vi "Acquire Image.vi"(8 "error in (no error)":errorcluster, 11 "Simulated Camera in":refnum<class "Simulated Camera.lvclass">) -> (0 "error out":errorcluster, 3 "Simulated Camera out":refnum<class "Simulated Camera.lvclass">)   [LabVIEW 2019, in "Simulated Camera.lvclass"]
uses:
  Simulated Camera.lvclass
  Simulated Camera.lvclass/Simulated Camera.ctl
  <vilib>/numeric/Random Number (Range) U64.vi
  <vilib>/numeric/sub_Random U32.vi
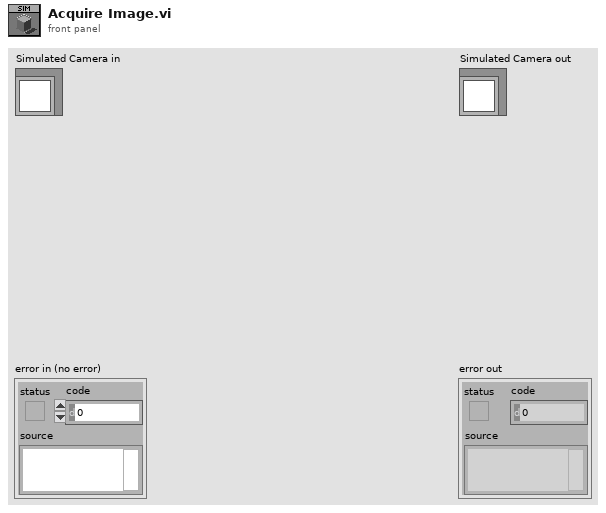
[diagram p1: front panel]
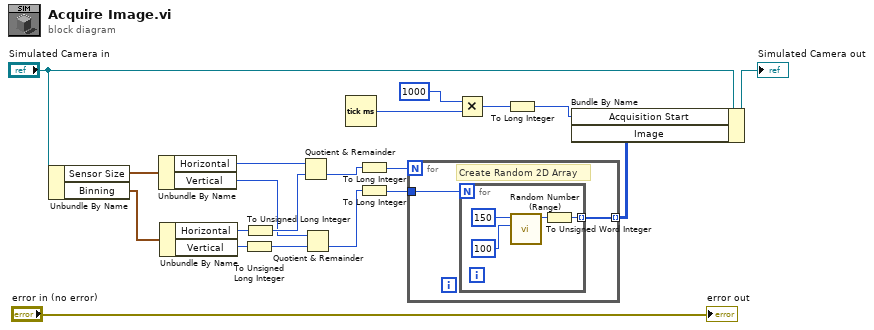
[diagram p0: block diagram]
diagram:
  n1 = Unbundle By Name("Simulated Camera in") -> ("Sensor Size"=w17:cluster{"Horizontal":u32, "Vertical":u32}, "Binning"=w16:cluster{"Horizontal":u16, "Vertical":u16})
  n2 = Unbundle By Name(w17) -> ("Horizontal"=w15:u32, "Vertical"=w10:u32)
  n3 = Unbundle By Name(w16) -> ("Horizontal"=w14:u16, "Vertical"=w12:u16)
  n4 = To Unsigned Long Integer(number=w12) -> (unsigned 32bit integer=w11:u32)
  n5 = To Unsigned Long Integer(number=w14) -> (unsigned 32bit integer=w13:u32)
  n6 = Quotient & Remainder(x=w15, y=w13) -> (floor(x/y)=w6:u32)  [unwired: 1 out]
  n7 = Quotient & Remainder(x=w10, y=w11) -> (floor(x/y)=w7:u32)  [unwired: 1 out]
  n8 = Tick Count (ms)() -> (millisecond timer value=w4:u32)
  n9 = To Long Integer(number=w6) -> (32bit integer=w9:i32)
  n10 = To Long Integer(number=w7) -> (32bit integer=w8:i32)
  n11 = for {
    N: w9 -> [_]
    tunnel: [w22] -> w5 mode=indexing
    tunnel: w8 -> [w21]
    # "Create Random 2D Array"
    n12 = for {
      N: w21 -> [_]
      tunnel: [w25] -> w22 mode=indexing
      n13 = call-poly <vilib>:"Random Number (Range).vi"("lower bound (0)"=u64 100, "upper bound (100)"=u64 150) -> ("number"=w26:u64)  [unwired: 9 in]
      n14 = To Unsigned Word Integer(number=w26) -> (unsigned 16bit integer=w25:u16)
    }
  }
  n15 = Multiply(x=u32 1000, y=w4) -> (x*y=w2:u32)
  n16 = To Long Integer(number=w2) -> (32bit integer=w1:i32)
  n17 = Bundle By Name(cluster="Simulated Camera in", "Acquisition Start"=w1, "Image"=w5) -> (→"Simulated Camera out":refnum<class "Simulated Camera.lvclass">)
  "error out" <- "error in (no error)"
